vi "F Dwf Analog In Status Sample.vi"(8 "error in (no error)":errorcluster, 9 "pdVoltSample":dbl, 10 "idxChannel":i32, 11 "hdwf":i32) -> (0 "error out":errorcluster, 1 "pdVoltSample out":dbl, 3 "function return":i32)   [LabVIEW 2019, in "Olasdwf.lvlib"]
doc: "DWFAPI int FDwfAnalogInStatusSample(HDWF hdwf, int idxChannel, double *pdVoltSample);"
uses:
  Olasdwf.lvlib
  Windows/System32/dwf.dll
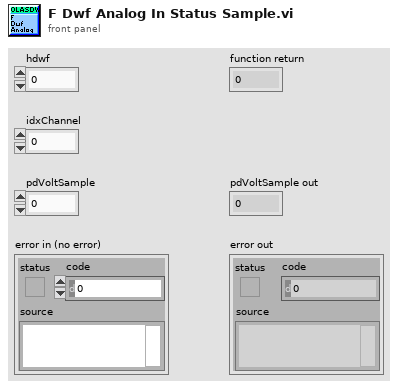
[diagram p1: front panel]
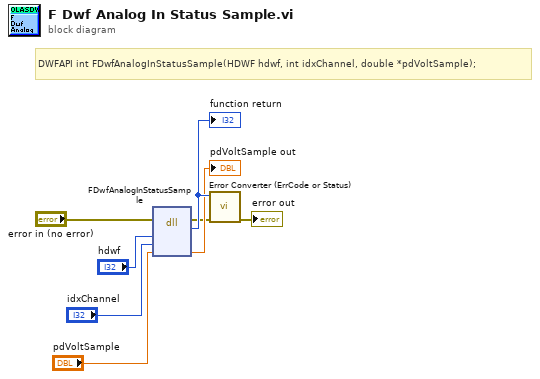
[diagram p0: block diagram]
diagram:
  # "DWFAPI int FDwfAnalogInStatusSample(HDWF hdwf, int idxChannel, double *pdVoltSample);"
  n1 = dll-call lib="C:/Windows/System32/dwf.*" fn="FDwfAnalogInStatusSample"(error in="error in (no error)", "hdwf"="hdwf", "idxChannel"="idxChannel", "pdVoltSample"="pdVoltSample") -> (error out=w2:errorcluster, w8:i32, "pdVoltSample"=→"pdVoltSample out":dbl)  [unwired: 4 in, 1 out]
  "function return" <- w8
  n2 = call "Error Converter (ErrCode or Status).vi"("error in (no error)"=w2, "error code"=w8) -> ("error out"=→"error out":errorcluster)  [unwired: 9 in]
